vi "MRC Smart IO Get Digital Input.vi"(8 "error in (no error)":errorcluster, 11 "deviceIndex":i32) -> (0 "error out":errorcluster, 2 "value out":u8)   [LabVIEW 2026, in "MrcLib.lvlib"]
doc: "MRC_Status MRC_CALLCONV MRC_SmartIO_GetDigitalInput(int32_t deviceIndex, MRC_Bool* value);"
uses:
  MrcLib.lvlib
  MrcLib.so
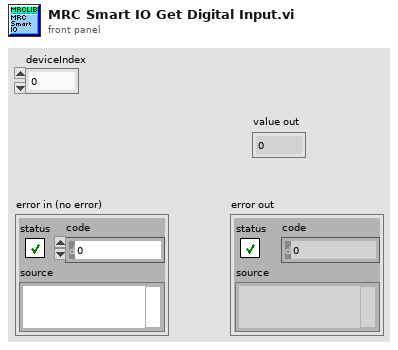
[diagram p1: front panel]
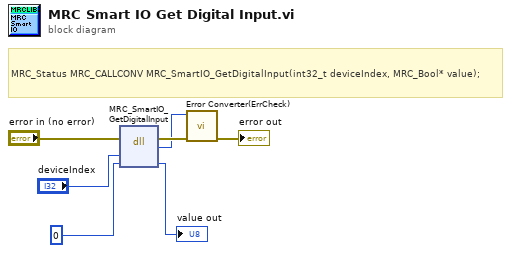
[diagram p0: block diagram]
diagram:
  # "MRC_Status MRC_CALLCONV MRC_SmartIO_GetDigitalInput(int32_t deviceIndex, MRC_Bool* value);"
  n1 = dll-call lib="MrcLib.*" fn="MRC_SmartIO_GetDigitalInput"(error in="error in (no error)", "deviceIndex"="deviceIndex", "value"=u8 0 ("value out")) -> (error out=w4:errorcluster, "return type"=w2:i32, "value"=→"value out":u8)  [unwired: 3 in, 1 out]
  n2 = call "Error Converter(ErrCheck).vi"("error in (no error)"=w4, "status"=w2) -> ("error out"=→"error out":errorcluster)  [unwired: 9 in]
